vi "UShortToLittleEndian.vi"(9 "Number":u16=1000) -> (1 "byte array":u8[](array[numeric]) format="%x")   [LabVIEW 2009]
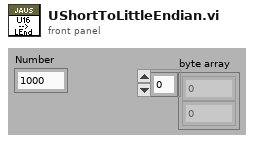
[diagram p1: front panel]
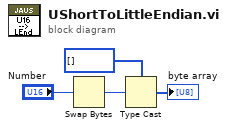
[diagram p0: block diagram]
diagram:
  n1 = Swap Bytes(anything="Number") -> (byte swapped=w3:u16)
  n2 = Type Cast(type=u8[] [], x=w3) -> (*(type *) &x=→"byte array":u8[])
